vi "Find_Current_Floor.vi"(8 "error in (no error)":errorcluster, 9 "Floors":T1, 10 "Elevator Status in":T2={"Door"=enum."Closed", "Person"=enum."Occupied", "Floors"={"0"=FALSE, "1"=FALSE, "2"=FALSE, "3"=FALSE}, "Up/Down/Idle"=enum."Idle", "Car Calls for Each Floor"=[FALSE, FALSE, FALSE, FALSE], "Up/Down Hall Calls for Each Floor"=[[{FALSE}, {FALSE}], [{FALSE}, {FALSE}], [{FALSE}, {FALSE}], [{FALSE}, {FALSE}], [{FALSE}, {FALSE}]], "ID"=0, "Start Timestamp"=0, "Target Duration"=0.0}, 11 "Elevator Fleet in":T8) -> (0 "error out":errorcluster, 1 "Current Floor":i32, 2 "Elevator Status out":T2={"Door"=enum."Closed", "Person"=enum."Occupied", "Floors"={"0"=FALSE, "1"=FALSE, "2"=FALSE, "3"=FALSE}, "Up/Down/Idle"=enum."Idle", "Car Calls for Each Floor"=[FALSE, FALSE, FALSE, FALSE], "Up/Down Hall Calls for Each Floor"=[[{FALSE}, {FALSE}], [{FALSE}, {FALSE}], [{FALSE}, {FALSE}], [{FALSE}, {FALSE}], [{FALSE}, {FALSE}]], "ID"=0, "Start Timestamp"=0, "Target Duration"=0.0}, 3 "Elevator Fleet out":T8)   [LabVIEW 2026]
uses:
  Controls/Elevator_Fleet.ctl
  Controls/Elevator_Status.ctl
  Controls/Door_Status_Enum.ctl
  Controls/Occupy_Status.ctl
  Controls/Floor_Status.ctl
  Controls/Motion_Status_Enum.ctl
  Controls/Car_Calls_Status.ctl
  Controls/Hall_Calls_Status.ctl
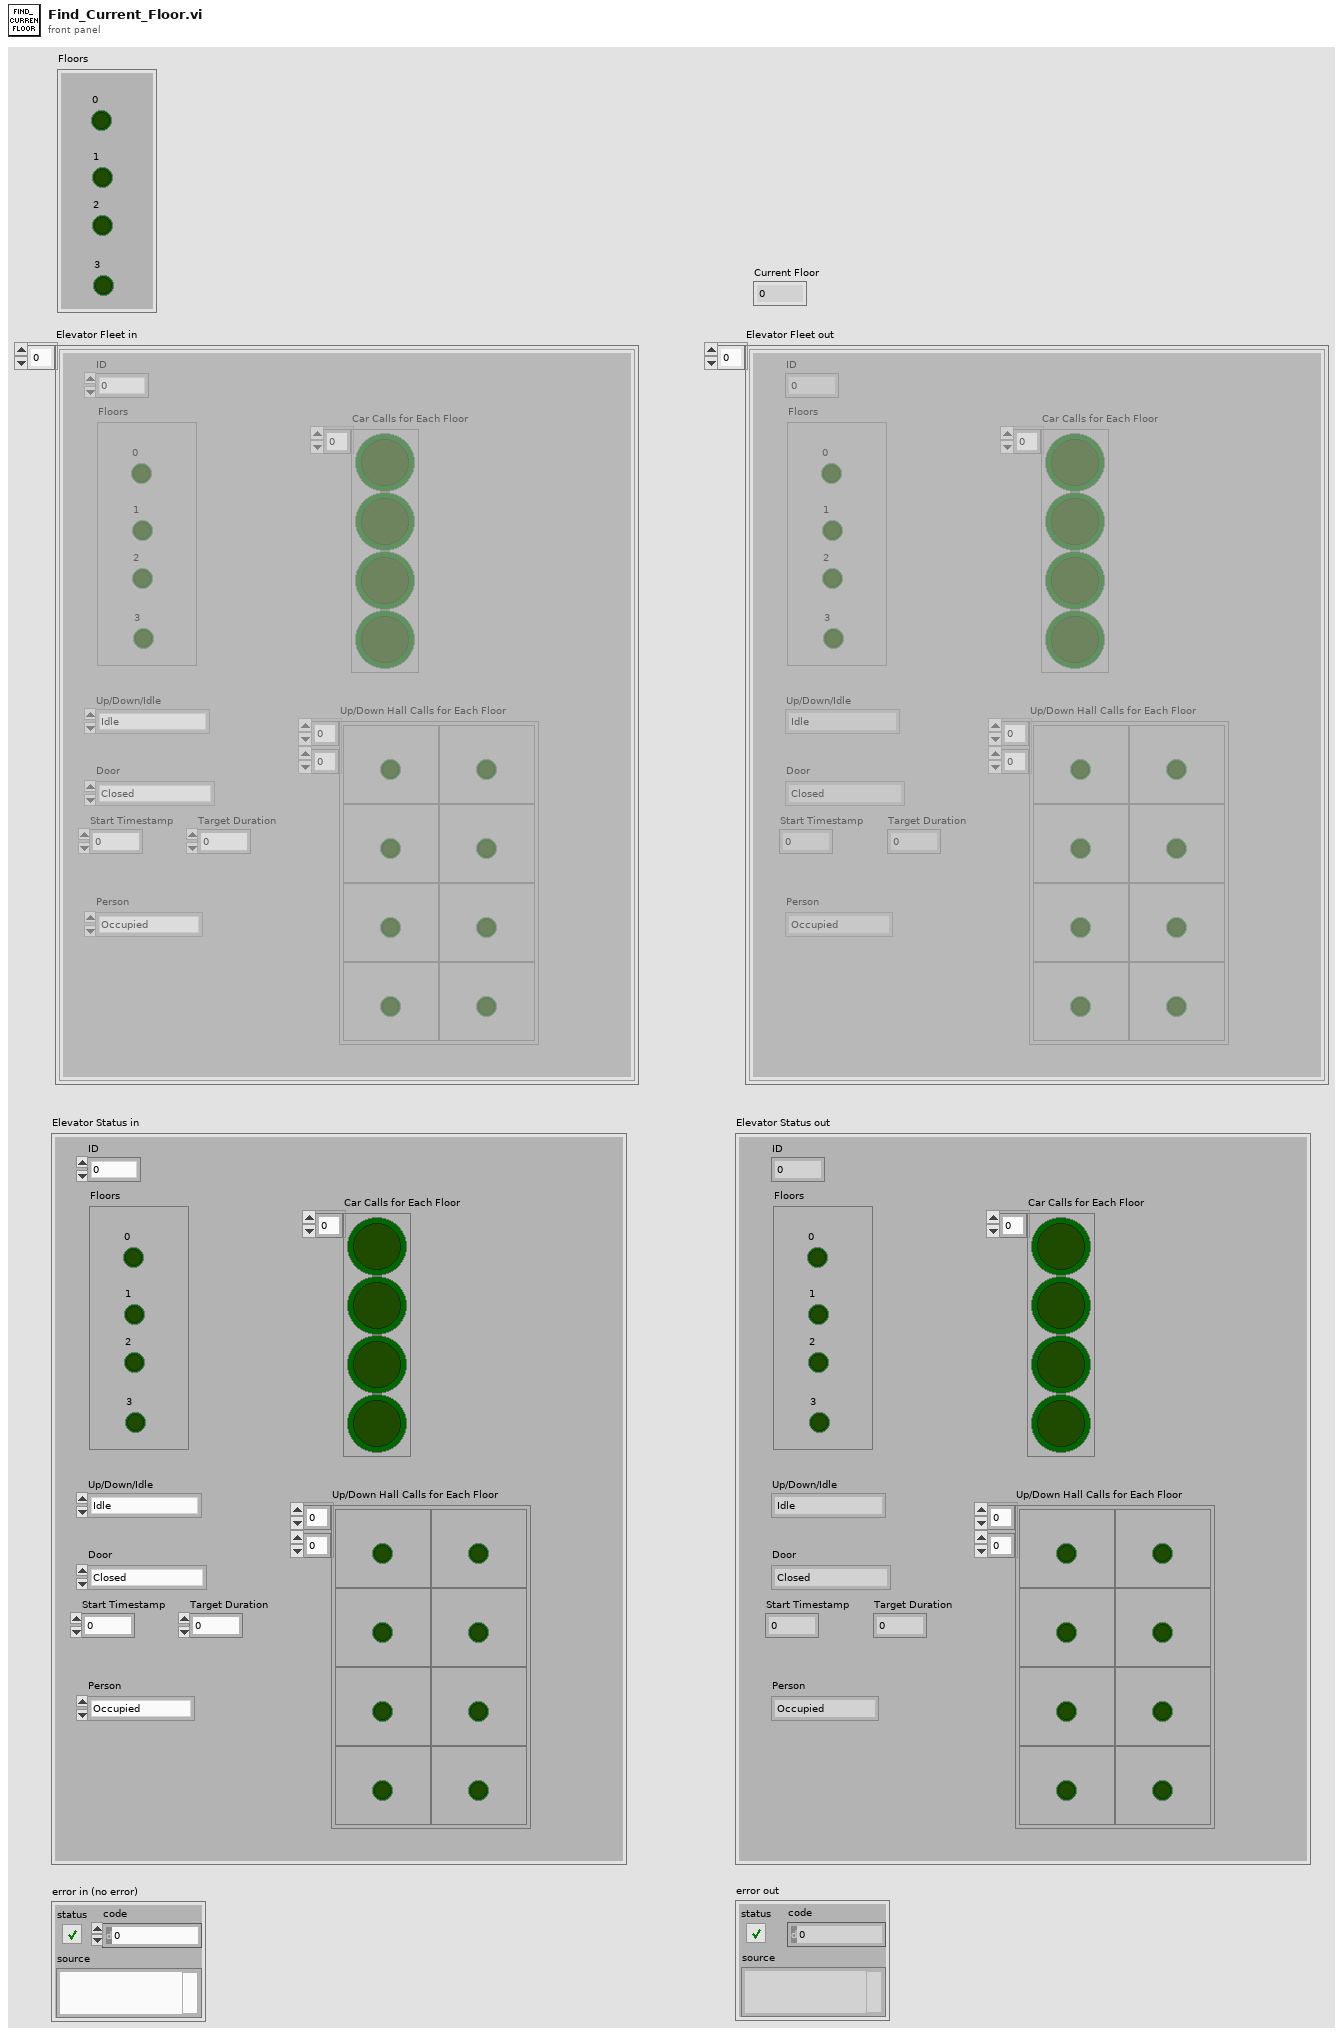
[diagram p1: front panel]
types:
  T1 = typedef "Floor_Status.ctl" = cluster{"0":bool, "1":bool, "2":bool, "3":bool}
  T2 = typedef "Elevator_Status.ctl" = cluster{"Door":T3, "Person":T4, "Floors":T1, "Up/Down/Idle":T5, "Car Calls for Each Floor":T6, "Up/Down Hall Calls for Each Floor":T7, "ID":i32, "Start Timestamp":u32, "Target Duration":dbl}
  T3 = typedef "Door_Status_Enum.ctl" = enum16{"Closed", "Open", "Opening", "Closing"}
  T4 = typedef "Occupy_Status.ctl" = enum16{"Occupied", "Empty"}
  T5 = typedef "Motion_Status_Enum.ctl" = enum16{"Idle", "Up", "Down"}
  T6 = typedef "Car_Calls_Status.ctl" = bool[]
  T7 = typedef "Hall_Calls_Status.ctl" = cluster{bool}[][]
  T8 = typedef "Elevator_Fleet.ctl" = T2[]
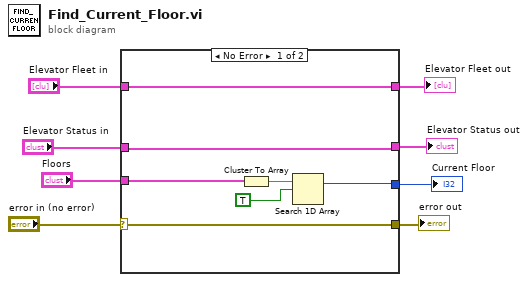
[diagram p0: block diagram]
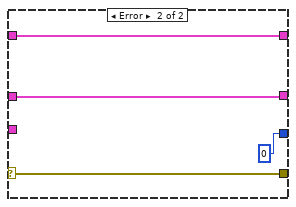
[diagram p2: hidden frame]
diagram:
  n1 = case shown="No Error" "error in (no error)" {
    selector: "error in (no error)" -> [w12 w19]
    tunnel: [w15 0 ("index of element")] -> w8
    tunnel: [w12 w19] -> w6
    tunnel: "Elevator Status in" -> [w9 w16]
    tunnel: "Elevator Fleet in" -> [w11 w17]
    tunnel: [w9 w16] -> w3
    tunnel: [w11 w17] -> w2
    tunnel: "Floors" -> [w10 _]
    frame No Error {
      n2 = Cluster To Array(cluster=w10) -> (array=w14:bool[])
      n3 = Search 1D Array(1D array=w14, element=TRUE ("0")) -> (index of element=w15:i32)  [unwired: 1 in]
    }
    frame Error {
    }
  }
  "Current Floor" <- w8
  "error out" <- w6
  "Elevator Fleet out" <- w2
  "Elevator Status out" <- w3
